vi "WinCI Convert Cfg String.vi"(7 "conversion action":T1, 9 "project details in":T2, 11 "config data in":string) -> (1 "config data out":string, 3 "project details out":T2)   [LabVIEW 2017, in "NI_SCC_WinCI.lvlib"]
uses:
  <vilib>/SourceControl/Providers/WinCI/NI_SCC_WinCI.lvlib
  <vilib>/SourceControl/Providers/WinCI/WinCI SCC Project Details.ctl
  <vilib>/SourceControl/support/SCCSup ConfigData Conv.ctl
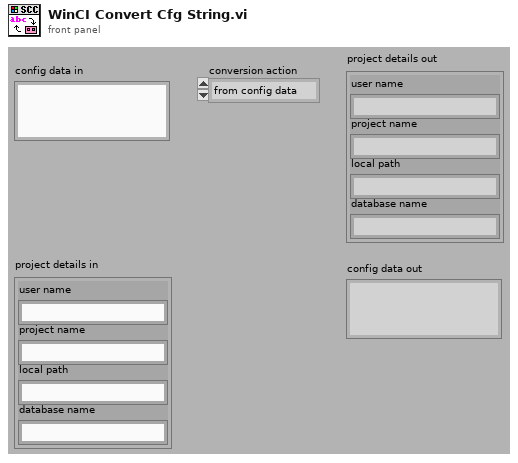
[diagram p1: front panel]
types:
  T1 = typedef "SCCSup ConfigData Conv.ctl" = enum16{"from config data", "to config data"}
  T2 = typedef "NI_SCC_WinCI.lvlib/WinCI SCC Project Details.ctl" = cluster{"user name":string, "project name":string, "local path":string, "database name":string}
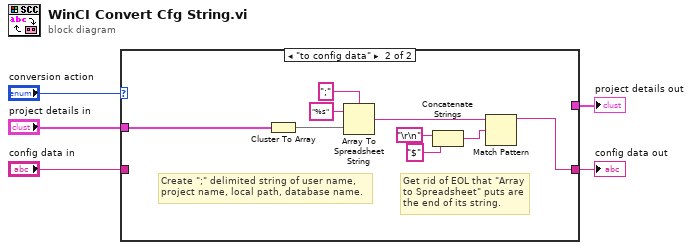
[diagram p0: block diagram]
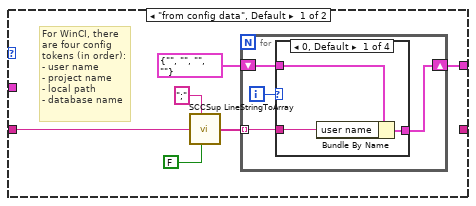
[diagram p2: hidden frame]
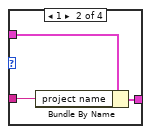
[diagram p3: hidden frame]
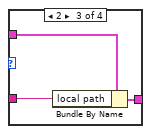
[diagram p4: hidden frame]
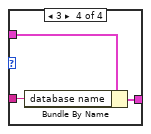
[diagram p5: hidden frame]
diagram:
  n1 = case shown="\"to config data\"" "conversion action" {
    tunnel: "config data in" -> [w7 _]
    tunnel: "project details in" -> [_ w36]
    tunnel: [w10 _] -> w2
    tunnel: [_ w28] -> w1
    frame "from config data", Default {
      # "For WinCI, there are four config tokens (in order):\n- user name\n- project name\n- local path\n- database name"
      n2 = call <vilib>:"SCCSup LineStringToArray.vi"("delimiter (Tab)"=";", "line string"=w7, "remove last empty element? (T)"=FALSE) -> ("line array"=w6:string[])  [unwired: 6 out]
      n3 = for {
        tunnel: w6 -> [w14] mode=indexing
        shift-right: [w12] -> w10
        shift-left: T2 {"user name"="", "project name"="", "local path"="", "database name"=""} ("project details in") -> [w13]
        i -> [w15]
        n4 = case shown="0, Default" w15 {
          tunnel: w14 -> [w17 w20 w23 w26]
          tunnel: w13 -> [w18 w21 w24 w27]
          tunnel: [w16 w19 w22 w25] -> w12
          frame 0, Default {
            n5 = Bundle By Name(cluster=w18, "user name"=w17) -> (w16:T2)
          }
          frame 1 {
            n6 = Bundle By Name(cluster=w21, "project name"=w20) -> (w19:T2)
          }
          frame 2 {
            n7 = Bundle By Name(cluster=w24, "local path"=w23) -> (w22:T2)
          }
          frame 3 {
            n8 = Bundle By Name(cluster=w27, "database name"=w26) -> (w25:T2)
          }
        }
      }
    }
    frame "to config data" {
      # "Get rid of EOL that \"Array to Spreadsheet\" puts are the end of its string."
      # "Create \";\" delimited string of user name, project name, local path, database name."
      n9 = Cluster To Array(cluster=w36) -> (array=w35:string[])
      n10 = Array To Spreadsheet String(delimiter (Tab)=";", array=w35, 3:"%s" ("format string")) -> (spreadsheet string=w32:string)
      n11 = Concatenate Strings("\r\n", "$" ("string")) -> (w29:string)
      n12 = Match Pattern(string=w32, regular expression=w29) -> (before substring=w28:string)  [unwired: 4 out]
    }
  }
  "project details out" <- w2
  "config data out" <- w1
